vi "Definition Cluster.vi"(11 "Double in":refnum<class "Double.lvclass">) -> (2 "Definition":variant, 3 "Double out":refnum<class "Double.lvclass">)   [LabVIEW 2020, in "Conditum.lvlib" / "Columns.lvlib" / "Double.lvclass"]
uses:
  Double.lvclass
  Double.lvclass/Double.ctl
  Type/Type.lvclass
  Definition.ctl
  Type/Definition.ctl
  Attributes.ctl
  Conditum.lvlib
  Double Definition.ctl
  C:/dev/lv20CE/lv-conditum/Conditum/Columns/Type/Type.lvclass
  C:/dev/lv20CE/lv-conditum/Conditum/Columns/Double/Double.lvclass
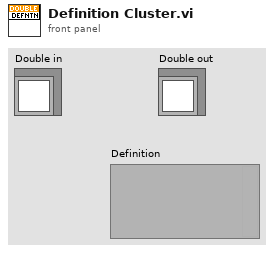
[diagram p1: front panel]
types:
  T1 = typedef "Conditum.lvlib/Columns.lvlib/Double.lvclass/Double Definition.ctl" = cluster{"Type":T2, "Attributes":T3, "Double":T4}
  T2 = typedef "Conditum.lvlib/Columns.lvlib/Type.lvclass/Definition.ctl" = cluster{"Name":string, "Nullable":bool, "Default NULL":bool}
  T3 = typedef "Conditum.lvlib/Attributes.ctl" = cluster{"Primary Key":bool, "Unique":bool, "Foreign Key":bool, "Auto Increment":bool}
  T4 = typedef "Conditum.lvlib/Columns.lvlib/Double.lvclass/Definition.ctl" = cluster{"Default":dbl}
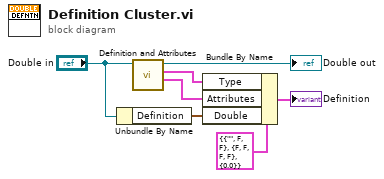
[diagram p0: block diagram]
diagram:
  n1 = Unbundle By Name("Double in") -> ("Definition"=w6:T4)
  n2 = call "Definition and Attributes.vi"("Type in"="Double in") -> ("Attributes"=w4:T3, "Definition"=w5:T2, "Type out"=→"Double out":refnum<class "Double.lvclass">)  [unwired: 8 in]
  n3 = Bundle By Name(cluster=T1 {"Type"={"Name"="", "Nullable"=FALSE, "Default NULL"=FALSE}, "Attributes"={"Primary Key"=FALSE, "Unique"=FALSE, "Foreign Key"=FALSE, "Auto Increment"=FALSE}, "Double"={"Default"=0.0}} ("Double Definition"), "Type"=w5, "Attributes"=w4, "Double"=w6) -> (→"Definition":T1)
